vi "Global 1.vi"() -> ()   [LabVIEW 2017]
panel:
  in  "Temp2":string
  in  "Temp1":string
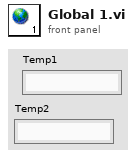
[diagram p1: front panel]
diagram:
